vi "LoadSSF_DSF.vi"(11 "SF_PATH":string) -> (0 "下段因子数据":dbl[][](array[numeric]), 1 "因子棒号":string[](array[string]), 2 "SF_0K":bool, 3 "上段因子数据":dbl[][](array[numeric]), 5 "文件INFO":string)   [LabVIEW 2020]
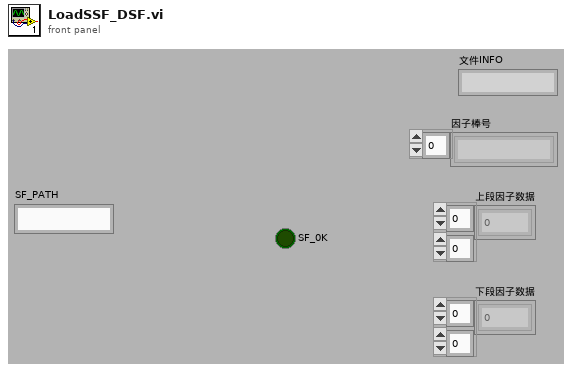
[diagram p1: front panel]
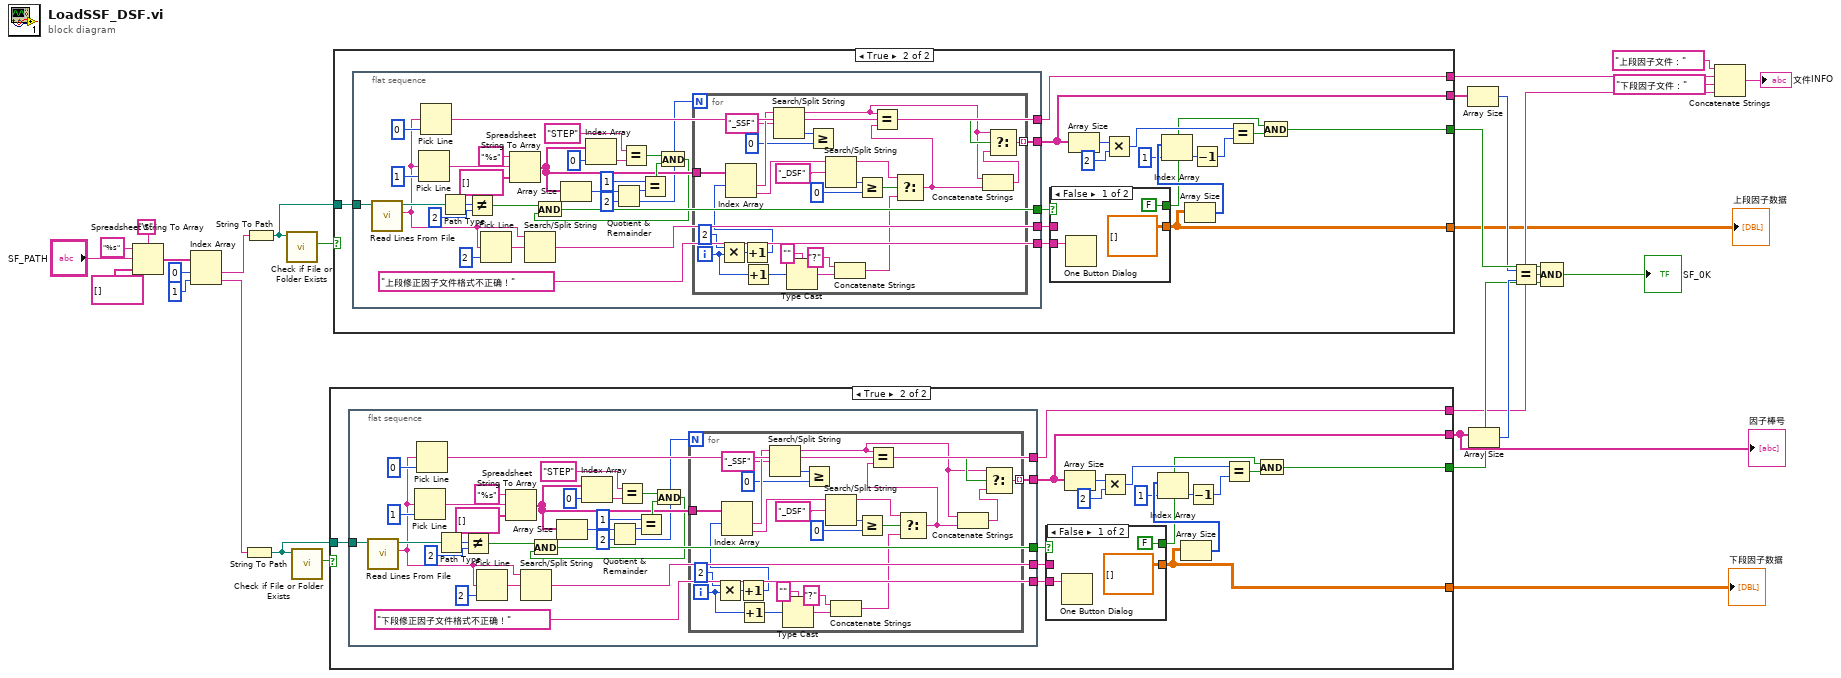
[diagram p0: block diagram]
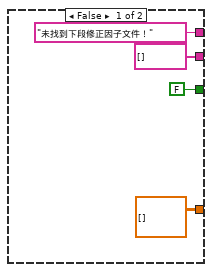
[diagram p2: hidden frame]
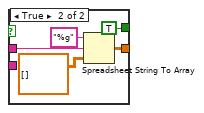
[diagram p3: hidden frame]
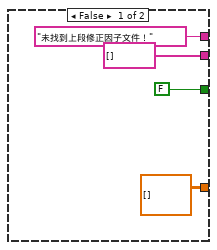
[diagram p4: hidden frame]
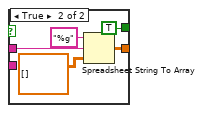
[diagram p5: hidden frame]
diagram:
  n1 = Spreadsheet String To Array(delimiter (Tab)="\t", format string="%s", spreadsheet string="SF_PATH", array type (2D Dbl)=string[] [] ("添加的数组")) -> (array=w22:string[])
  n2 = Index Array(array=w22, index #1=0 ("index"), index #2=1 ("index")) -> (element #1=w6:string, element #2=w5:string)
  n3 = String To Path(string=w5) -> (path=w3:path)
  n4 = String To Path(string=w6) -> (path=w4:path)
  n5 = call <vilib>:"Check if File or Folder Exists.vi"("path"=w4) -> ("file or folder exists?"=w28:bool)  [unwired: 8 in, 2 out]
  n6 = call <vilib>:"Check if File or Folder Exists.vi"("path"=w3) -> ("file or folder exists?"=w20:bool)  [unwired: 8 in, 2 out]
  n7 = case shown="True" w20 {
    tunnel: [dbl[][] [] ("type (empty)") w33] -> w1
    tunnel: w3 -> [_ w46]
    tunnel: [FALSE ("file or folder exists?") w36] -> w15
    tunnel: ["未找到下段修正因子文件！" ("output string") w35] -> w7
    tunnel: [string[] [] w34] -> w18
    frame False {
    }
    frame True {
      n8 = flat-sequence {
        tunnel: [w75] -> w49
        tunnel: [w67] -> w48
        tunnel: ["下段修正因子文件格式不正确！" ("消息")] -> w47
        tunnel: w46 -> [w72]
        tunnel: [w66] -> w35
        tunnel: [w51] -> w34
        frame #0 {
          n9 = call <vilib>:"Read Lines From File.vi"("file path (dialog if empty)"=w72) -> ("new file path (Not A Path if cancelled)"=w74:path, "line string"=w68:string)  [unwired: 5 in, 2 out]
          n10 = Pick Line ("选行并添加至字符串")(multi-line string=w68, line index=1 ("行索引")) -> (output string=w64:string)  [unwired: 1 in]
          n11 = Pick Line ("选行并添加至字符串")(multi-line string=w68, line index=0 ("行索引")) -> (output string=w66:string)  [unwired: 1 in]
          n12 = Path Type(1:w74) -> (0:w78:i16)
          n13 = Not Equal?(x=w78, y=i16 2) -> (x != y?=w76:bool)
          n14 = Pick Line ("选行并添加至字符串")(multi-line string=w68, line index=2 ("行索引")) -> (output string=w69:string)  [unwired: 1 in]
          n15 = Spreadsheet String To Array ("电子表格字符串至数组转换")(format string="%s" ("format (%.3f)"), spreadsheet string=w64, array type (2D Dbl)=string[] [] ("添加的数组")) -> (array=w53:string[])  [unwired: 1 in]
          n16 = Search/Split String(string=w68, search string/char (-)=w69) -> (match + rest of string=w67:string)  [unwired: 1 in, 2 out]
          n17 = Array Size(array=w53) -> (size(s)=w59:i32)
          n18 = Index Array(array=w53, index=0 ("索引")) -> (element=w61:string)
          n19 = Quotient & Remainder(x=w59, y=2) -> (x-y*floor(x/y)=w57:i32, floor(x/y)=w52:i32)
          n20 = Equal?(x="STEP", y=w61) -> (x = y?=w54:bool)
          n21 = Equal?(x=1, y=w57) -> (x = y?=w55:bool)
          n22 = And(x=w54, y=w55) -> (x .and. y?=w50:bool)
          n23 = And(x=w76, y=w50) -> (x .and. y?=w75:bool)
          n24 = for {
            N: w52 -> [_]
            tunnel: w53 -> [w104]
            tunnel: [w88] -> w51 mode=indexing
            i -> [w90]
            n25 = Multiply(x=2, y=w90) -> (x*y=w102:i32)
            n26 = Increment(x=w102) -> (x+1=w101:i32)
            n27 = Index Array(array=w104, index #1=w101) -> (element #1=w100:string, element #2=w93:string)  [unwired: 1 in]
            n28 = Increment(x=w90) -> (x+1=w89:i32)
            n29 = Search/Split String(string=w100, search string/char (-)="_SSF" ("搜索字符串/字符(-)")) -> (substring before match=w83:string, offset of match=w98:i32)  [unwired: 1 in, 1 out]
            n30 = Type Cast(type="" ("类型"), x=w89) -> (*(type *) &x=w87:string)
            n31 = Greater Or Equal?(x=w98, y=0) -> ()  [unwired: 1 out]
            n32 = Search/Split String(string=w93, search string/char (-)="_DSF" ("搜索字符串/字符(-)")) -> (substring before match=w85:string, offset of match=w95:i32)  [unwired: 1 in, 1 out]
            n33 = Concatenate Strings("?" ("字符串"), w87) -> (w82:string)
            n34 = Greater Or Equal?(x=w95, y=0) -> (x >= y?=w80:bool)
            n35 = Select(t=w85, s=w80, f=w82) -> (s? t:f=w81:string)
            n36 = Equal?(x=w83, y=w81) -> (x = y?=w92:bool)
            n37 = Concatenate Strings(w83, w81) -> (w84:string)
            n38 = Select(t=w83, s=w92, f=w84) -> (s? t:f=w88:string)
          }
        }
      }
      n39 = case shown="False" w49 {
        tunnel: w48 -> [_ w109]
        tunnel: [dbl[][] [] ("type (empty)") w110] -> w33
        tunnel: w47 -> [w106 _]
        tunnel: [FALSE ("file or folder exists?") TRUE ("file or folder exists?")] -> w37
        frame False {
          n40 = One Button Dialog(message=w106) -> ()  [unwired: 1 in, 1 out]
        }
        frame True {
          n41 = Spreadsheet String To Array ("电子表格字符串至数组转换")(format string="%g" ("format (%.3f)"), spreadsheet string=w109, array type (2D Dbl)=dbl[][] [] ("type (empty)")) -> (array=w110:dbl[][])  [unwired: 1 in]
        }
      }
      n42 = Array Size(array=w34) -> (size(s)=w42:i32)
      n43 = Multiply(x=w42, y=2) -> (x*y=w40:i32)
      n44 = Array Size(array=w33) -> (size(s)=w45:i32[])
      n45 = Index Array(array=w45, index=1 ("索引")) -> (element=w43:i32)
      n46 = Decrement(x=w43) -> (x-1=w39:i32)
      n47 = Equal?(x=w40, y=w39) -> (x = y?=w38:bool)
      n48 = And(x=w37, y=w38) -> (x .and. y?=w36:bool)
    }
  }
  "因子棒号" <- w18
  "下段因子数据" <- w1
  n49 = case shown="True" w28 {
    tunnel: w4 -> [_ w130]
    tunnel: [FALSE ("file or folder exists?") w120] -> w16
    tunnel: ["未找到上段修正因子文件！" ("output string") w119] -> w10
    tunnel: [string[] [] w118] -> w19
    tunnel: [dbl[][] [] ("type (empty)") w117] -> w2
    frame False {
    }
    frame True {
      n50 = flat-sequence {
        tunnel: [w159] -> w133
        tunnel: [w151] -> w132
        tunnel: ["上段修正因子文件格式不正确！" ("消息")] -> w131
        tunnel: w130 -> [w156]
        tunnel: [w150] -> w119
        tunnel: [w135] -> w118
        frame #0 {
          n51 = call <vilib>:"Read Lines From File.vi"("file path (dialog if empty)"=w156) -> ("new file path (Not A Path if cancelled)"=w158:path, "line string"=w152:string)  [unwired: 5 in, 2 out]
          n52 = Pick Line ("选行并添加至字符串")(multi-line string=w152, line index=1 ("行索引")) -> (output string=w148:string)  [unwired: 1 in]
          n53 = Pick Line ("选行并添加至字符串")(multi-line string=w152, line index=0 ("行索引")) -> (output string=w150:string)  [unwired: 1 in]
          n54 = Path Type(1:w158) -> (0:w162:i16)
          n55 = Not Equal?(x=w162, y=i16 2) -> (x != y?=w160:bool)
          n56 = Pick Line ("选行并添加至字符串")(multi-line string=w152, line index=2 ("行索引")) -> (output string=w153:string)  [unwired: 1 in]
          n57 = Spreadsheet String To Array ("电子表格字符串至数组转换")(format string="%s" ("format (%.3f)"), spreadsheet string=w148, array type (2D Dbl)=string[] [] ("添加的数组")) -> (array=w137:string[])  [unwired: 1 in]
          n58 = Search/Split String(string=w152, search string/char (-)=w153) -> (match + rest of string=w151:string)  [unwired: 1 in, 2 out]
          n59 = Array Size(array=w137) -> (size(s)=w143:i32)
          n60 = Index Array(array=w137, index=0 ("索引")) -> (element=w145:string)
          n61 = Quotient & Remainder(x=w143, y=2) -> (x-y*floor(x/y)=w141:i32, floor(x/y)=w136:i32)
          n62 = Equal?(x="STEP", y=w145) -> (x = y?=w138:bool)
          n63 = Equal?(x=1, y=w141) -> (x = y?=w139:bool)
          n64 = And(x=w138, y=w139) -> (x .and. y?=w134:bool)
          n65 = And(x=w160, y=w134) -> (x .and. y?=w159:bool)
          n66 = for {
            N: w136 -> [_]
            tunnel: w137 -> [w188]
            tunnel: [w172] -> w135 mode=indexing
            i -> [w174]
            n67 = Multiply(x=2, y=w174) -> (x*y=w186:i32)
            n68 = Increment(x=w186) -> (x+1=w185:i32)
            n69 = Index Array(array=w188, index #1=w185) -> (element #1=w184:string, element #2=w177:string)  [unwired: 1 in]
            n70 = Increment(x=w174) -> (x+1=w173:i32)
            n71 = Search/Split String(string=w184, search string/char (-)="_SSF" ("搜索字符串/字符(-)")) -> (substring before match=w167:string, offset of match=w182:i32)  [unwired: 1 in, 1 out]
            n72 = Type Cast(type="" ("类型"), x=w173) -> (*(type *) &x=w171:string)
            n73 = Greater Or Equal?(x=w182, y=0) -> ()  [unwired: 1 out]
            n74 = Search/Split String(string=w177, search string/char (-)="_DSF" ("搜索字符串/字符(-)")) -> (substring before match=w169:string, offset of match=w179:i32)  [unwired: 1 in, 1 out]
            n75 = Concatenate Strings("?" ("字符串"), w171) -> (w166:string)
            n76 = Greater Or Equal?(x=w179, y=0) -> (x >= y?=w164:bool)
            n77 = Select(t=w169, s=w164, f=w166) -> (s? t:f=w165:string)
            n78 = Equal?(x=w167, y=w165) -> (x = y?=w176:bool)
            n79 = Concatenate Strings(w167, w165) -> (w168:string)
            n80 = Select(t=w167, s=w176, f=w168) -> (s? t:f=w172:string)
          }
        }
      }
      n81 = case shown="False" w133 {
        tunnel: w132 -> [_ w193]
        tunnel: [dbl[][] [] ("type (empty)") w194] -> w117
        tunnel: w131 -> [w190 _]
        tunnel: [FALSE ("file or folder exists?") TRUE ("file or folder exists?")] -> w121
        frame False {
          n82 = One Button Dialog(message=w190) -> ()  [unwired: 1 in, 1 out]
        }
        frame True {
          n83 = Spreadsheet String To Array ("电子表格字符串至数组转换")(format string="%g" ("format (%.3f)"), spreadsheet string=w193, array type (2D Dbl)=dbl[][] [] ("type (empty)")) -> (array=w194:dbl[][])  [unwired: 1 in]
        }
      }
      n84 = Array Size(array=w118) -> (size(s)=w126:i32)
      n85 = Multiply(x=w126, y=2) -> (x*y=w124:i32)
      n86 = Array Size(array=w117) -> (size(s)=w129:i32[])
      n87 = Index Array(array=w129, index=1 ("索引")) -> (element=w127:i32)
      n88 = Decrement(x=w127) -> (x-1=w123:i32)
      n89 = Equal?(x=w124, y=w123) -> (x = y?=w122:bool)
      n90 = And(x=w121, y=w122) -> (x .and. y?=w120:bool)
    }
  }
  "上段因子数据" <- w2
  n91 = Array Size(array=w19) -> (size(s)=w13:i32)
  n92 = Array Size(array=w18) -> (size(s)=w17:i32)
  n93 = Equal?(x=w13, y=w17) -> (x = y?=w12:bool)
  n94 = Compound Arithmetic op=AND(w16, w12, w15) -> (→"SF_0K":bool)
  n95 = Concatenate Strings("上段因子文件：" ("字符串"), w10, "下段因子文件：" ("字符串"), w7) -> (→"文件INFO":string)
